vi "CommonSig-Apply Ramp (1D).vi"(0 "Array in":dbl[](array[numeric]), 5 "Ramp up (ms)":dbl=5.0, 7 "Ramp down (ms)":dbl=5.0, 9 "Fs (Hz)":dbl, 11 "error in (no error)":errorcluster, 12 "Asymmetric":bool) -> (4 "Array out":dbl[](array[numeric]), 15 "error out":errorcluster)   [LabVIEW 2020]
uses:
  Classes/Gate/Shape.ctl
  Classes/Gate/Gate.lvclass/Gate.ctl
  00fa021d-ebe0-42e5-9c35-5538040c7da1.vi
  Classes/Gate/Write Ramp (ms).vi
  Classes/Gate/Write Down (ms).vi
  Classes/Gate/Write Asymmetric.vi
  Classes/Gate/Write Shape.vi
  Classes/Gate/Write Duration (ms).vi
  Classes/Gate/Gate.lvclass
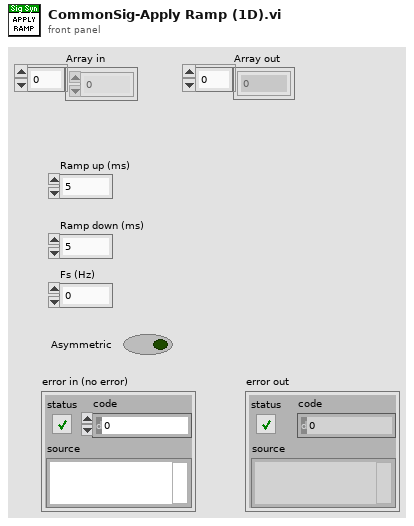
[diagram p1: front panel]
types:
  T1 = typedef "Gate.lvclass/Shape.ctl" = enum16{"OFF", "Rectangle", "Sine-squared", "Trapezoid"}
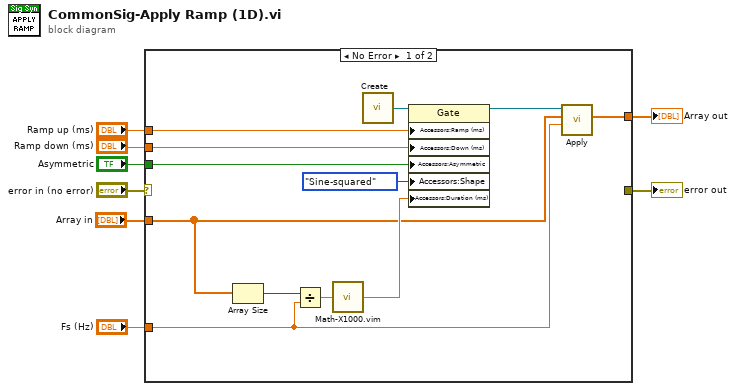
[diagram p0: block diagram]
diagram:
  n1 = case shown="No Error" "error in (no error)" {
    selector: "error in (no error)" -> [_ w21]
    tunnel: "Ramp up (ms)" -> [w20 _]
    tunnel: "Array in" -> [w10 w22]
    tunnel: [w16 w22] -> w6
    tunnel: "Fs (Hz)" -> [w17 _]
    tunnel: "Ramp down (ms)" -> [w19 _]
    tunnel: "Asymmetric" -> [w18 _]
    tunnel: [_ w21] -> w1
    frame No Error {
      n2 = Array Size(array=w10) -> (size(s)=w9:i32)
      n3 = Divide(x=w9, y=w17) -> (x/y=w12:dbl)
      n4 = call "Math-X1000.vim"("X"=w12) -> ("1000X"=w11:dbl)
      n5 = call "Create.vi"() -> ("Gate"=w15:refnum<class "Gate.lvclass">)  [unwired: 15 in]
      n6 = property class="Gate"(reference=w15, "Accessors:Ramp (ms)"=w20, "Accessors:Down (ms)"=w19, "Accessors:Asymmetric"=w18, "Accessors:Shape"=Shape."Sine-squared" ("Shape"), "Accessors:Duration (ms)"=w11) -> (reference out=w14:refnum<class "Gate.lvclass">)  [unwired: 1 in, 1 out]
      n7 = call "Apply.vi"("Fs (Hz)"=w17, "Array in"=w10, "Gate in"=w14) -> ("Array out"=w16:dbl[])  [unwired: 6 in, 2 out]
    }
    frame Error {
    }
  }
  "Array out" <- w6
  "error out" <- w1
